vi "esp301 set backlash.vi"(7 "Seperator in":string, 8 "error in (no error)":errorcluster, 9 "Args":string[](array[string]), 10 "String":string, 11 "ESP301 in":refnum<class "ESP301.lvclass">) -> (0 "error out":errorcluster, 2 "new commands":string, 3 "ESP301 out":refnum<class "ESP301.lvclass">)   [LabVIEW 2020, in "ESP301.lvclass"]
uses:
  ESP301.lvclass
  ESP301.lvclass/ESP301.ctl
  shared/CompressAndUpdate(Poly)/CompressAndUpdate(Numeric).vi
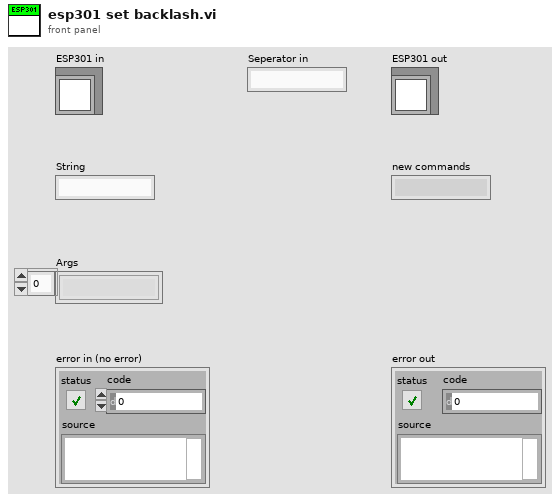
[diagram p1: front panel]
types:
  T1 = cluster{"Axis 1":cluster{"Value":dbl, "Min":dbl, "Max":dbl, "StepSize":dbl, "Tolerance":dbl, "ValueActual":dbl}, "Axis 2":cluster{"Value":dbl, "Min":dbl, "Max":dbl, "StepSize":dbl, "Tolerance":dbl, "ValueActual":dbl}, "Axis 3":cluster{"Value":dbl, "Min":dbl, "Max":dbl, "StepSize":dbl, "Tolerance":dbl, "ValueActual":dbl}}
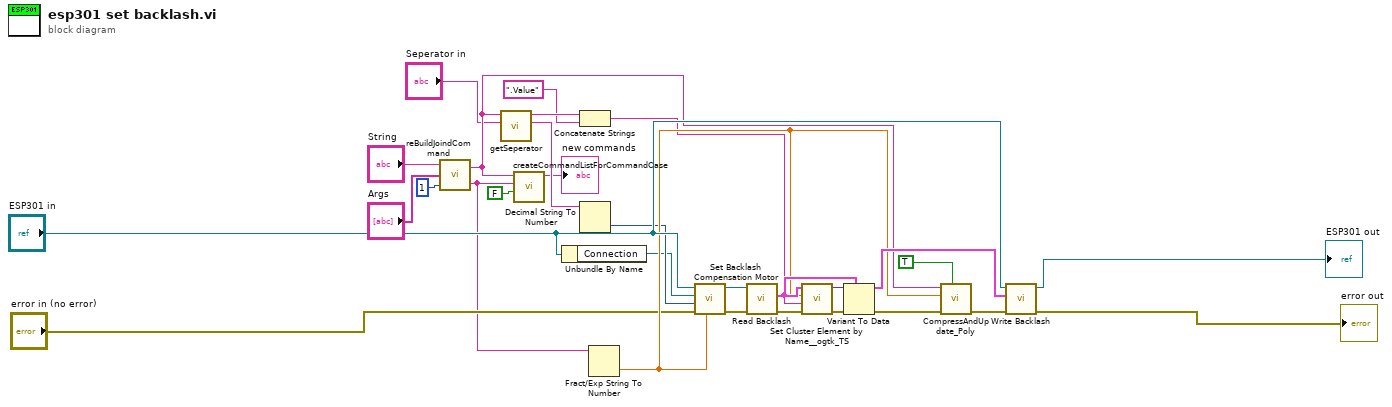
[diagram p0: block diagram]
diagram:
  n1 = call "reBuildJoindCommand.vi"("number of group elements (0)"=1, "Args"="Args", "Command 2"="String") -> ("Arg"=w12:string, "Command"=w16:string)
  n2 = call "getSeperator.vi"("Channel Seperator (\"\")"="Seperator in", "Command"=w16) -> ("Channel"=w8:string, "Seperator (e.g. \"Channel1\")"=w10:string)  [unwired: 8 in]
  n3 = call "createCommandListForCommandCase.vi"("immediate Check (only once)"=FALSE, "setvalue"=w12, "command"=w16) -> ("new commands"=→"new commands":string)  [unwired: 8 in]
  n4 = Unbundle By Name("ESP301 in") -> ("Connection"=w18:refnum<visa-resource-name>)
  n5 = Concatenate Strings(w10, ".Value" ("string")) -> (w11:string)
  n6 = Decimal String To Number(string=w8) -> (number=w19:i32)  [unwired: 2 in, 1 out]
  n7 = Fract/Exp String To Number(string=w12) -> (number=w20:dbl)  [unwired: 3 in, 1 out]
  n8 = call-dynamic "Set Backlash Compensation Motor.vi"("Backlash Compensation Value (0 units)"=w20, "error in (no error)"="error in (no error)", "Axis (1)"=w19, "VISA resource name"=w18, "ESP301 in"="ESP301 in") -> ("error out"=w24:errorcluster, "ESP301 out"=w22:refnum<class "ESP301.lvclass">)  [unwired: 4 in, 1 out]
  n9 = call "Read Backlash.vi"("error in (no error)"=w24, "ESP301 in"=w22) -> ("error out"=w25:errorcluster, "Backlash"=w23:T1)  [unwired: 7 in, 1 out]
  n10 = call "Set Cluster Element by Name__ogtk_TS.vi"("error in (no error)"=w25, "Element Name (\"\": New Element Data Name)"=w11, "New Element Value"=w20, "Cluster"=w23) -> ("error out"=w13:errorcluster, "VCluster out"=w14:variant)  [unwired: 5 in, 1 out]
  n11 = Variant To Data(error in=w13, type=w23, Variant=w14) -> (data=w27:T1, error out=w15:errorcluster)
  n12 = call-poly "CompressAndUpdate_Poly.vi"("force CVT update (false)"=TRUE ("force CVT update"), "error in"=w15, "Numeric"=w20, "command or variable name"=w16) -> ("error out"=w28:errorcluster)  [unwired: 7 in]
  n13 = call "Write Backlash.vi"("error in (no error)"=w28, "Backlash"=w27, "ESP301 in"="ESP301 in") -> ("error out"=→"error out":errorcluster, "ESP301 out"=→"ESP301 out":refnum<class "ESP301.lvclass">)  [unwired: 7 in]
